vi "GoalProbabilityDensity.vi"(11 "IA state":T1={"our_robots"=[], "enemy_robots"=[], "balls"=[], "geometry"={"line_width"=0, "field_length"=0, "field_width"=0, "boundary_width"=0, "referee_width"=0, "goal_width"=0, "goal_depth"=0, "goal_wall_width"=0, "center_circle_radius"=0, "defense_radius"=0, "defense_stretch"=0, "free_kick_from_defense_dist"=0, "penalty_spot_from_field_line_dist"=0, "penalty_line_from_spot_dist"=0}, "IA Judge"={"stage"="", "command"="", "our_goalie_id"=0.0, "enemy_goalie_id"=0.0, "command enum"=enum."Halt", "Time"=enum."Azul"}, "Received Timestamp"=timestamp(0 s since 1904-01-01), "Events"={"Touch"=FALSE, "Ball out"=FALSE, "id touch"=0.0, "Ball out of \nVision"=FALSE, "Ball inside \nGoalie area"=FALSE, "Robot not responding"=FALSE, "Robots responding status"=[1.0, 1.0, 1.0, 1.0, 1.0, 1.0], "Enemy Ball \nPossession"=FALSE, "Pass State"=FALSE, "id end of pass"=0.0, "Kick"=FALSE, "Id ini Possession"=0.0, "Ball Possesion"=FALSE, "Id Possesion"=0.0}}) -> (3 "2D Probability Matrix":dbl[][](array[numeric]))   [LabVIEW 2017]
uses:
  Intel/Functions Enum.ctl
  Intel/AttackerStates.ctl
  Core/AI Robot.ctl
  Core/AI Ball.ctl
  Core/Field Size.ctl
  Intel/Command Enum.ctl
  Core/AI Judge.ctl
  Util/Events/Events.ctl
  Core/AI Input.ctl
panel:
  out "grid x out":dbl format="%#_13g"
  out "grid y out":dbl format="%#_13g"
  in  "grid y":dbl=30.0 format="%#_13g"
  in  "grid x":dbl=45.0 format="%#_13g"
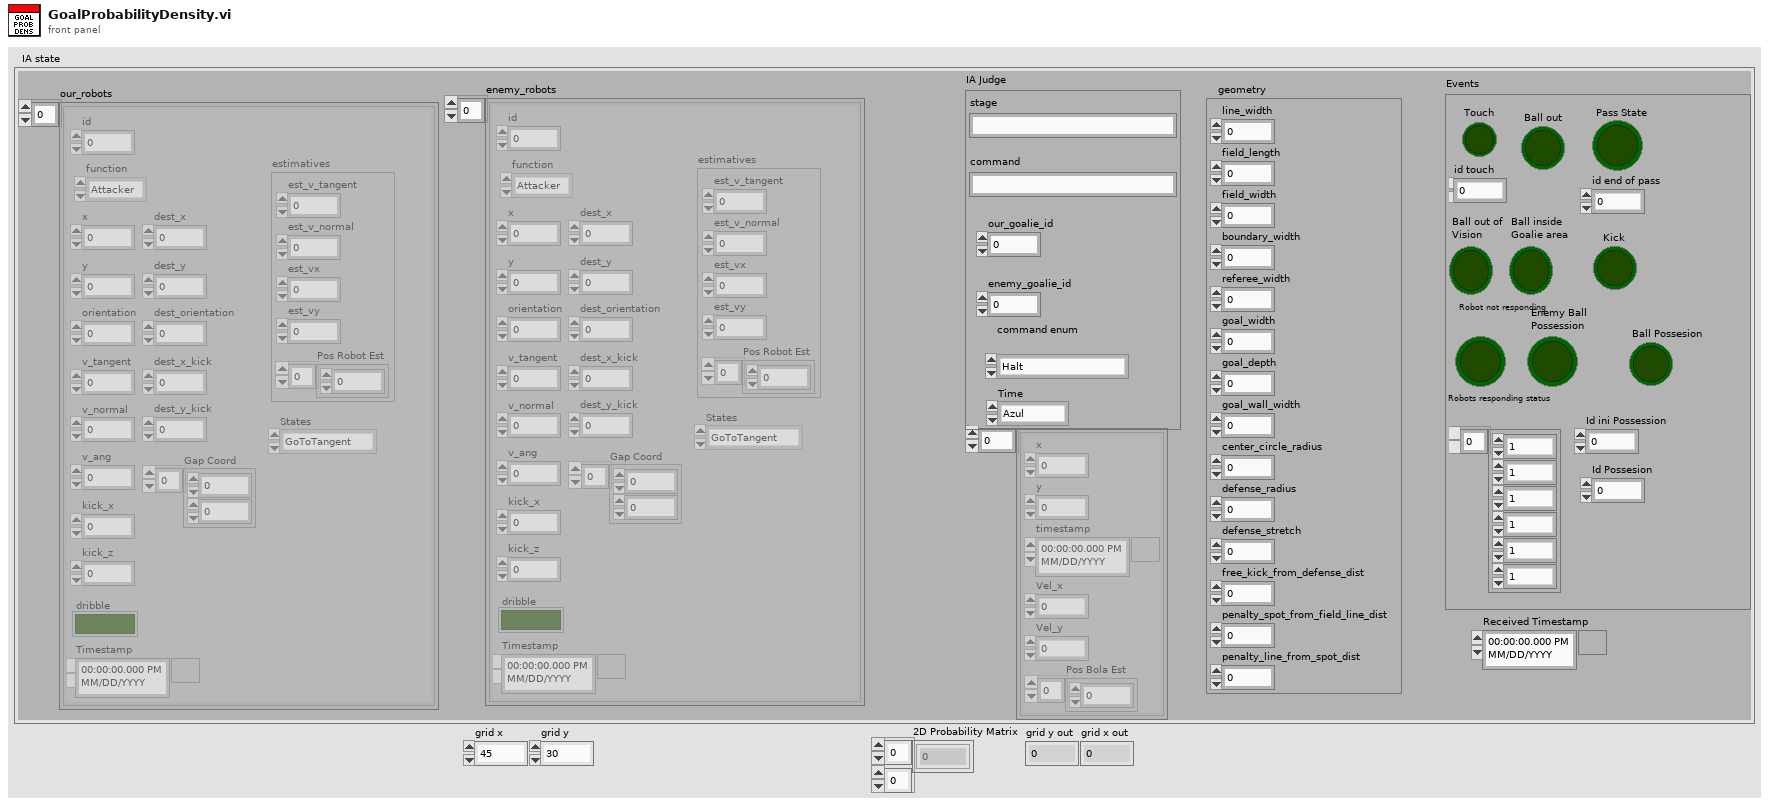
[diagram p1: front panel]
types:
  T1 = typedef "AI Input.ctl" = cluster{"our_robots":T2[], "enemy_robots":T2[], "balls":T5[], "geometry":T6, "IA Judge":T7, "Received Timestamp":timestamp, "Events":T9}
  T2 = typedef "AI Robot.ctl" = cluster{"id":u32, "function":T3, "x":dbl, "y":dbl, "orientation":dbl, "v_tangent":dbl, "v_normal":dbl, "v_ang":dbl, "kick_x":dbl, "kick_z":dbl, "dribble":bool, "Timestamp":timestamp, "dest_x":dbl, "dest_y":dbl, "dest_orientation":dbl, "estimatives":cluster{"est_v_tangent":dbl, "est_v_normal":dbl, "est_vx":dbl, "est_vy":dbl, "Pos Robot Est":dbl[]}, "dest_x_kick":dbl, "dest_y_kick":dbl, "Gap Coord":dbl[], "States":T4}
  T3 = typedef "Functions Enum.ctl" = enum16{"Attacker", "Goalie", "Defender", "Striker", "Goto 0", "Dummy", "Kicker", "ZigZag"}
  T4 = typedef "AttackerStates.ctl" = enum16{"Pass", "GoToTangent", "BallGetting", "GoToKick", ""}
  T5 = typedef "AI Ball.ctl" = cluster{"x":dbl, "y":dbl, "timestamp":timestamp, "Vel_x":dbl, "Vel_y":dbl, "Pos Bola Est":dbl[]}
  T6 = typedef "Field Size.ctl" = cluster{"line_width":u32, "field_length":u32, "field_width":u32, "boundary_width":u32, "referee_width":u32, "goal_width":u32, "goal_depth":u32, "goal_wall_width":u32, "center_circle_radius":u32, "defense_radius":u32, "defense_stretch":u32, "free_kick_from_defense_dist":u32, "penalty_spot_from_field_line_dist":u32, "penalty_line_from_spot_dist":u32}
  T7 = typedef "AI Judge.ctl" = cluster{"stage":string, "command":string, "our_goalie_id":dbl, "enemy_goalie_id":dbl, "command enum":T8, "Time":enum16{"Azul", "Amarelo"}}
  T8 = typedef "Command Enum.ctl" = enum16{"Halt", "Stop", "Force Start", "PKA Normal Start", "Prepare Kickoff Ally", "PKE Normal Start", "Prepare Kickoff Enemy", "Prepare Penalty Ally", "PPA Normal Start", "Prepare Penalty Enemy", "PPE Normal Start", "Direct Free Enemy", "Direct Free Ally", "Indirect Free Enemy", "Indirect Free Ally", "Timeout Enemy", "Timeout Ally", "Goal Enemy", "Goal Ally", "Ball Placement Enemy", "Ball Placement Ally", "Normal Half Time", "Extra Time Break", "Extra Half Time", "None", "Post Game"}
  T9 = typedef "Events.ctl" = cluster{"Touch":bool, "Ball out":bool, "id touch":dbl, "Ball out of \nVision":bool, "Ball inside \nGoalie area":bool, "Robot not responding":bool, "Robots responding status":dbl[], "Enemy Ball \nPossession":bool, "Pass State":bool, "id end of pass":dbl, "Kick":bool, "Id ini Possession":dbl, "Ball Possesion":bool, "Id Possesion":dbl}
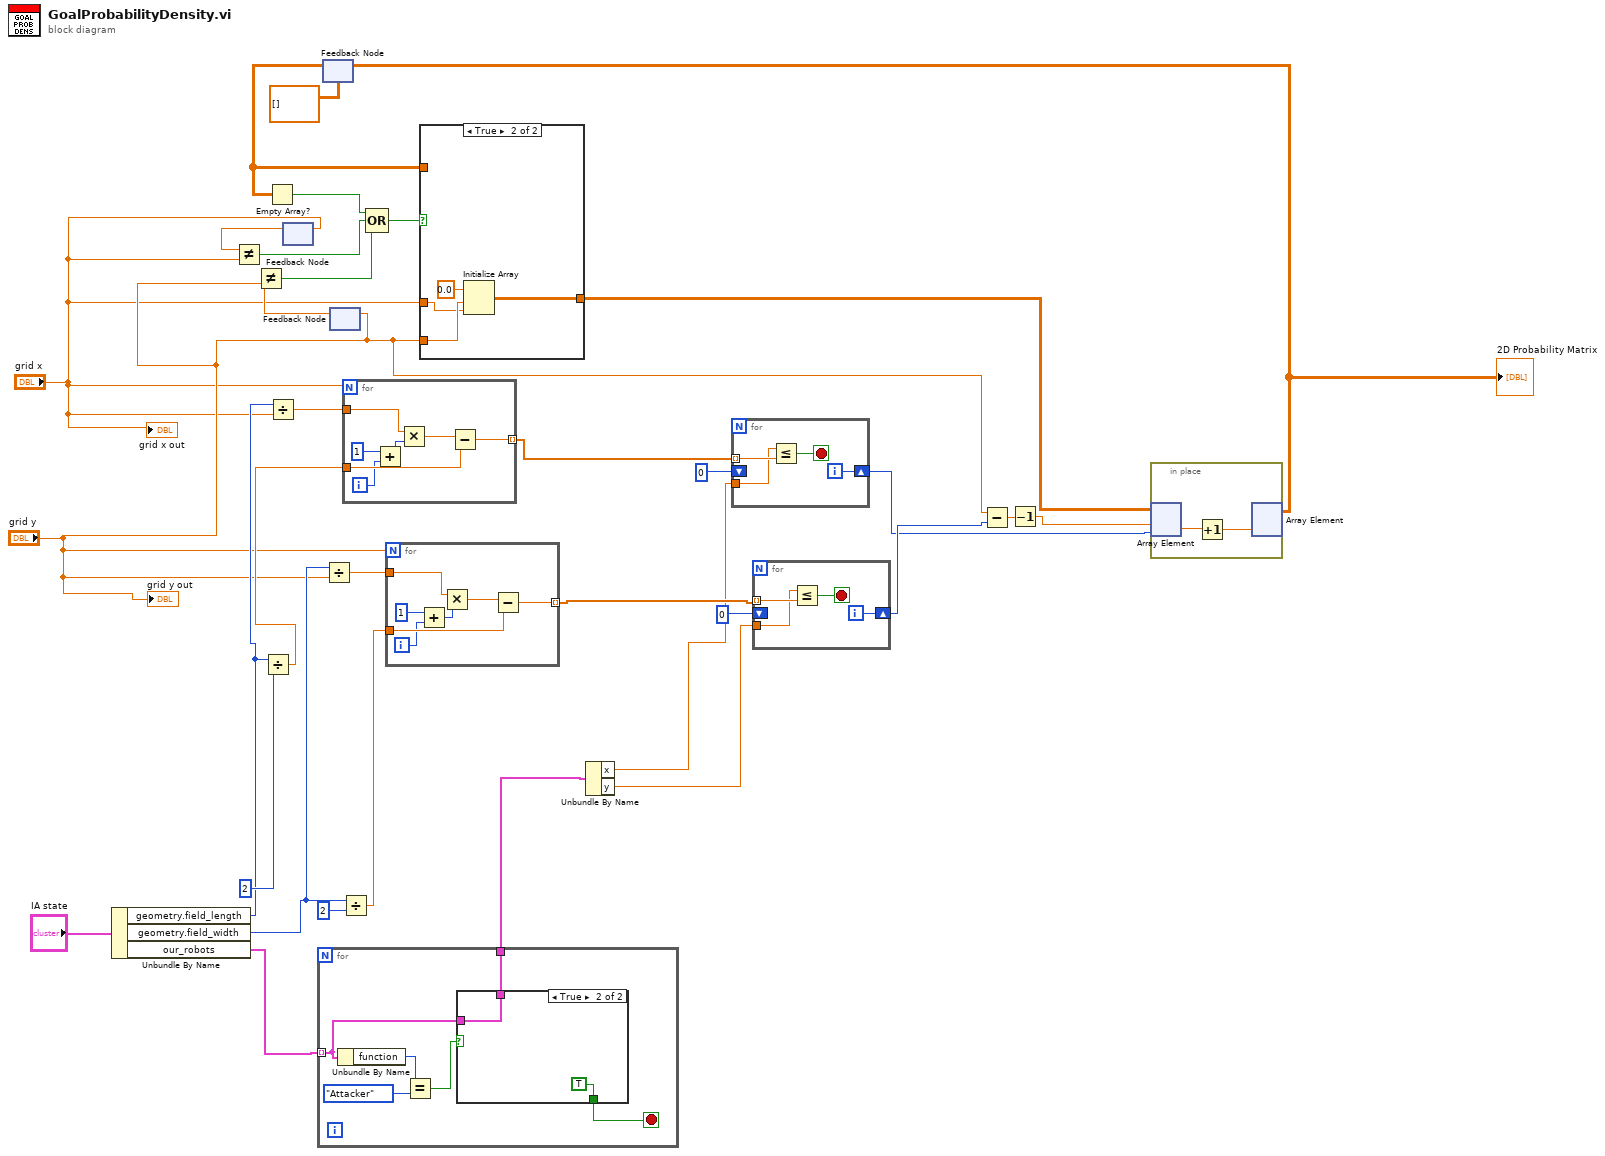
[diagram p0: block diagram]
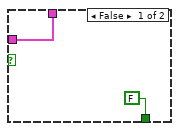
[diagram p2: hidden frame]
diagram:
  n1 = Unbundle By Name("IA state") -> ("geometry.field_length"=w29:u32, "geometry.field_width"=w28:u32, "our_robots"=w2:T2[])
  n2 = Divide(x=w29, y=u32 2) -> (x/y=w16:dbl)
  n3 = Divide(x=w29, y="grid x") -> (x/y=w26:dbl)
  n4 = feedback #1() -> (w25:dbl)  [unwired: 1 in]
  n5 = Not Equal?(x=w25, y="grid x") -> (x != y?=w22:bool)
  n6 = feedback-in #1("grid x") -> ()
  n7 = for {
    tunnel: w2 -> [w36] mode=indexing
    tunnel: [w35] -> w1
    stop <- w34 stop-if-true
    n8 = Unbundle By Name(w36) -> ("function"=w39:T3)
    n9 = Equal?(x=w39, y=Functions_Enum."Attacker") -> (x = y?=w37:bool)
    n10 = case shown="True" w37 {
      tunnel: w36 -> [w41 w43]
      tunnel: [w41 w43] -> w35
      tunnel: [FALSE TRUE] -> w34
      frame False {
      }
      frame True {
      }
    }
  }
  n11 = feedback #2(dbl[][] []) -> (w19:dbl[][])
  n12 = Empty Array?(array=w19) -> (empty?=w23:bool)
  n13 = Divide(x=w28, y="grid y") -> (x/y=w15:dbl)
  n14 = feedback #3() -> (w24:dbl)  [unwired: 1 in]
  n15 = Not Equal?(x=w24, y="grid y") -> (x != y?=w21:bool)
  n16 = feedback-in #3("grid y") -> ()
  n17 = Divide(x=w28, y=u32 2) -> (x/y=w30:dbl)
  n18 = for {
    N: "grid x" -> [_]
    tunnel: w26 -> [w50]
    tunnel: w16 -> [w47]
    tunnel: [w48] -> w13 mode=indexing
    i -> [w46]
    n19 = Add(x=1, y=w46) -> (x+y=w44:i32)
    n20 = Multiply(x=w50, y=w44) -> (x*y=w49:dbl)
    n21 = Subtract(x=w49, y=w47) -> (x-y=w48:dbl)
  }
  n22 = Compound Arithmetic op=OR(w23, w22, w21) -> (w20:bool)
  n23 = for {
    N: "grid y" -> [_]
    tunnel: w15 -> [w57]
    tunnel: w30 -> [w54]
    tunnel: [w55] -> w14 mode=indexing
    i -> [w53]
    n24 = Add(x=1, y=w53) -> (x+y=w52:i32)
    n25 = Multiply(x=w57, y=w52) -> (x*y=w56:dbl)
    n26 = Subtract(x=w56, y=w54) -> (x-y=w55:dbl)
  }
  n27 = case shown="True" w20 {
    tunnel: "grid x" -> [_ w59]
    tunnel: "grid y" -> [_ w60]
    tunnel: w19 -> [w58 _]
    tunnel: [w58 w61] -> w12
    frame False {
    }
    frame True {
      n28 = Initialize Array(0.0 ("element"), w60, w59) -> (w61:dbl[][])
    }
  }
  n29 = Unbundle By Name(w1) -> ("x"=w6:dbl, "y"=w5:dbl)
  n30 = for {
    shift-right: [w65] -> w9
    shift-left: 0 -> [_]
    tunnel: w13 -> [w64] mode=indexing
    tunnel: w6 -> [w63]
    i -> [w65]
    stop <- w66 stop-if-true
    n31 = Less Or Equal?(x=w63, y=w64) -> (x <= y?=w66:bool)
  }
  n32 = for {
    shift-right: [w69] -> w10
    shift-left: 0 -> [_]
    tunnel: w14 -> [w68] mode=indexing
    tunnel: w5 -> [w67]
    i -> [w69]
    stop <- w70 stop-if-true
    n33 = Less Or Equal?(x=w67, y=w68) -> (x <= y?=w70:bool)
  }
  n34 = Subtract(x="grid y", y=w10) -> (x-y=w8:dbl)
  n35 = Decrement(x=w8) -> (x-1=w7:dbl)
  n36 = in-place {
    n37 = in-place-array #4(w12, w7, w9) -> (w72:dbl)
    n38 = Increment(x=w72) -> (x+1=w71:dbl)
    n39 = in-place-array #4(w71) -> (w27:dbl[][])  [unwired: 2 out]
  }
  "2D Probability Matrix" <- w27
  n40 = feedback-in #2(w27) -> ()
  "grid y out" <- "grid y"
  "grid x out" <- "grid x"
